vi "Text to Picture Font Cluster.vi"(11 "Text Font Cluster":T1) -> (2 "Color":u32, 3 "Picture Font Cluster":T2)   [LabVIEW 2020, in "PieChart.lvclass"]
uses:
  PieChart.lvclass
  <vilib>/Utility/miscctls.llb/LVFontTypeDef.ctl
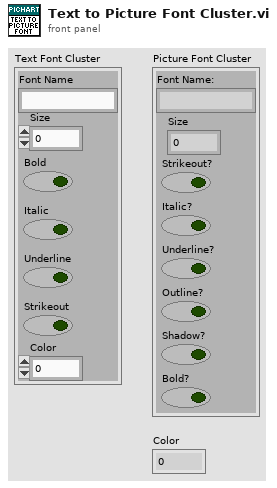
[diagram p1: front panel]
types:
  T1 = typedef "LVFontTypeDef.ctl" = cluster{"Font Name":string, "Size":u16, "Bold":bool, "Italic":bool, "Underline":bool, "Strikeout":bool, "Color":u32}
  T2 = cluster{"Font Name:":string, "Size":i16, "Strikeout?":bool, "Italic?":bool, "Underline?":bool, "Outline?":bool, "Shadow?":bool, "Bold?":bool}
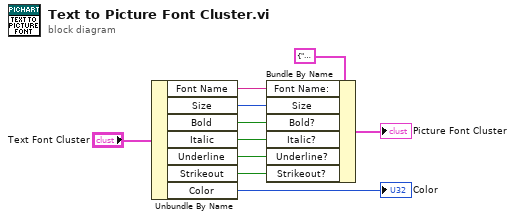
[diagram p0: block diagram]
diagram:
  n1 = Unbundle By Name("Text Font Cluster") -> ("Font Name"=w3:string, "Size"=w4:u16, "Bold"=w5:bool, "Italic"=w6:bool, "Underline"=w7:bool, "Strikeout"=w8:bool, "Color"=→"Color":u32)
  n2 = Bundle By Name(cluster=T2 {"Font Name:"="Arial", "Size"=15, "Strikeout?"=FALSE, "Italic?"=FALSE, "Underline?"=FALSE, "Outline?"=FALSE, "Shadow?"=FALSE, "Bold?"=FALSE} ("[user-specified font]"), "Font Name:"=w3, "Size"=w4, "Bold?"=w5, "Italic?"=w6, "Underline?"=w7, "Strikeout?"=w8) -> (→"Picture Font Cluster":T2)
